vi "TMCM351- stopflag.vi"(3 "错误输入":errorcluster caption="错误输入（无错误）", 4 "motor":u8(ring) items=["x", "y", "z"], 5 "com in":refnum<visa-resource-name>) -> (0 "错误输出":errorcluster, 2 "com out":refnum<visa-resource-name>)   [LabVIEW 2018]
uses:
  module_param.vi
panel:
  # "149 \n清零"
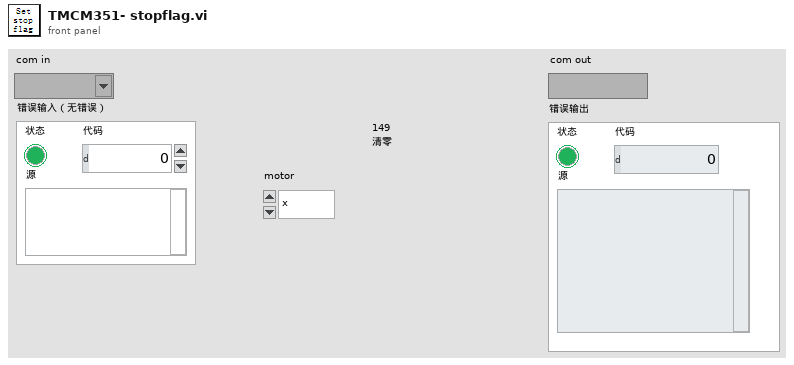
[diagram p1: front panel]
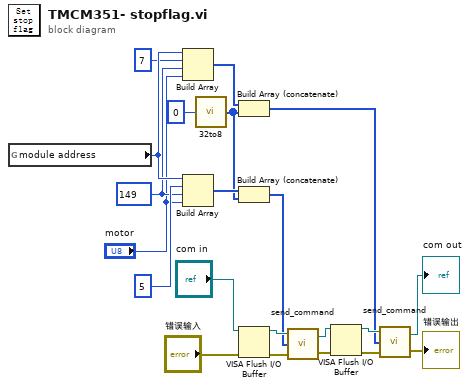
[diagram p0: block diagram]
diagram:
  w7 = u8 149
  n1 = global read "module_param.vi" "module address"() -> (w9:u8)
  n2 = Build Array(w9, u8 7 ("元素"), w7, "motor") -> (w5:u8[])
  n3 = Build Array(w9, u8 5, w7, "motor") -> (w16:u8[])
  n4 = call "32to8.vi"("32data_in"=0) -> ("8Array"=w4:u8[])
  n5 = Build Array (concatenate)(w5, w4) -> (w3:u8[])
  n6 = Build Array (concatenate)(w16, w4) -> (w15:u8[])
  n7 = VISA Flush I/O Buffer(VISA resource name="com in", error in (no error)="错误输入") -> (VISA resource name out=w18:refnum<visa-resource-name>, error out=w17:errorcluster)  [unwired: 1 in]
  n8 = call "send_command.vi"("错误输入"=w17, 3:w15, "com in"=w18) -> ("错误输出"=w10:errorcluster, "com out"=w11:refnum<visa-resource-name>)
  n9 = VISA Flush I/O Buffer(VISA resource name=w11, error in (no error)=w10) -> (VISA resource name out=w13:refnum<visa-resource-name>, error out=w12:errorcluster)  [unwired: 1 in]
  n10 = call "send_command.vi"("错误输入"=w12, 3:w3, "com in"=w13) -> ("错误输出"=→"错误输出":errorcluster, "com out"=→"com out":refnum<visa-resource-name>)
